vi "ParseSeriesID.vi"(8 "error in":errorcluster, 11 "json file path":path) -> (0 "error out":errorcluster, 1 "filename":string, 2 "owning folder":string, 3 "title":string)   [LabVIEW 2024]
uses:
  TypeDefs/series--cluster.ctl
  <vilib>/addons/_JKI.lib/Serialization/JSON/JKI JSON Serialization.lvlib
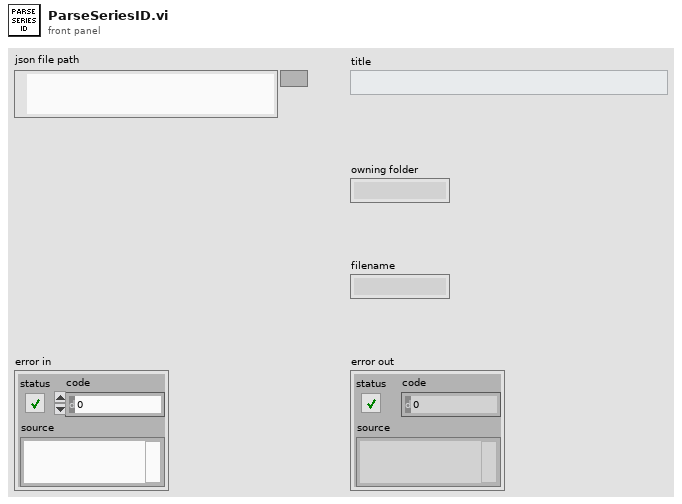
[diagram p1: front panel]
types:
  T1 = typedef "series--cluster.ctl" = cluster{"id":i32, "title":string, "description":string, "resourceURI":string, "urls":cluster{"type":string, "url":string}[], "startYear":i32, "endYear":i32, "rating":string, "type":string, "modified":variant, "thumbnail":cluster{"path":string, "extension":string}, "creators":cluster{"available":i32, "returned":i32, "collectionURI":string, "items":cluster{"resourceURI":string, "name":string, "role":string}[]}, "comics":cluster{"available":i32, "returned":i32, "collectionURI":string, "items":cluster{"resourceURI":string, "name":string}[]}, "characters":cluster{"available":i32, "returned":i32, "collectionURI":string, "items":cluster{"resourceURI":string, "name":string}[]}, "stories":cluster{"available":i32, "returned":i32, "collectionURI":string, "items":cluster{"resourceURI":string, "name":string, "type":string}[]}, "events":cluster{"available":i32, "returned":i32, "collectionURI":string, "items":cluster{"resourceURI":string, "name":string}[]}, "next":variant, "previous":variant}
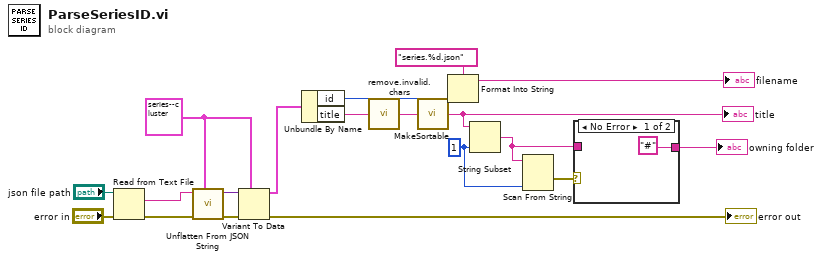
[diagram p0: block diagram]
diagram:
  w4 = 1 ("length (rest)")
  w12 = T1 {"id"=0, "title"="", "description"="", "resourceURI"="", "urls"=[], "startYear"=0, "endYear"=0, "rating"="", "type"="", "modified"=variant, "thumbnail"={"path"="", "extension"=""}, "creators"={"available"=0, "returned"=0, "collectionURI"="", "items"=[]}, "comics"={"available"=0, "returned"=0, "collectionURI"="", "items"=[]}, "characters"={"available"=0, "returned"=0, "collectionURI"="", "items"=[]}, "stories"={"available"=0, "returned"=0, "collectionURI"="", "items"=[]}, "events"={"available"=0, "returned"=0, "collectionURI"="", "items"=[]}, "next"=variant, "previous"=variant} ("Cluster")
  n1 = Read from Text File(file (use dialog)="json file path", error in="error in") -> (text=w17:string, error out=w16:errorcluster)  [unwired: 2 in, 2 out]
  n2 = call <vilib>:"Unflatten From JSON String.vi"("Type and Defaults"=w12, "error in (no error)"=w16, "JSON String"=w17) -> ("error out"=w14:errorcluster, "Variant"=w15:variant)  [unwired: 7 in]
  n3 = Variant To Data(error in=w14, type=w12, Variant=w15) -> (data=w13:T1, error out=→"error out":errorcluster)
  n4 = Unbundle By Name(w13) -> ("id"=w8:i32, "title"=w6:string)
  n5 = call "remove.invalid.chars.vi"("string in"=w6) -> ("string out"=w5:string)
  n6 = call "MakeSortable.vi"("string in"=w5) -> ("string out"=w11:string)
  "title" <- w11
  n7 = Format Into String(format string="series.%d.json", w8) -> (resulting string=→"filename":string)  [unwired: 2 in, 1 out]
  n8 = String Subset(string=w11, length (rest)=w4) -> (substring=w1:string)  [unwired: 1 in]
  n9 = Scan From String(input string=w1, default 1=w4) -> (error out=w3:errorcluster)  [unwired: 4 in, 2 out]
  n10 = case shown="No Error" w3 {
    tunnel: ["#" w21] -> w2
    tunnel: w1 -> [_ w21]
    frame No Error {
    }
    frame Default {
    }
  }
  "owning folder" <- w2
